vi "H_sub.vi"(4 "q 1":sgl[](array[numeric]), 5 "Id_in":i32, 6 "N 1":sgl[](array[numeric])) -> (0 "q":sgl[](array[numeric]), 2 "N":sgl[](array[numeric]))   [LabVIEW 2010]
panel:
  in  "Id_x":i32
  out "XY Graph":cluster{"q 1":sgl[], "N 1":sgl[]}[](graph)
  in  "qx":dbl
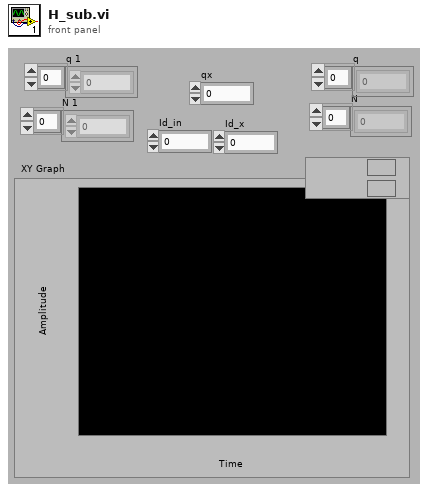
[diagram p1: front panel]
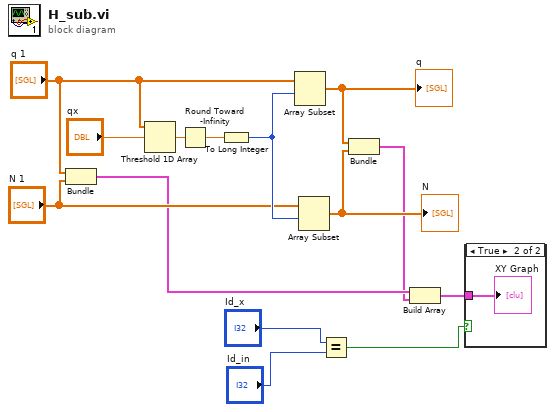
[diagram p0: block diagram]
diagram:
  n1 = Bundle("q 1"="q 1", "N 1"="N 1") -> (w6:cluster{"q 1":sgl[], "N 1":sgl[]})  [unwired: 1 in]
  n2 = Threshold 1D Array(2:"qx", 3:"q 1") -> (0:w13:sgl)  [unwired: 1 in]
  n3 = Round Toward -Infinity(1:w13) -> (0:w12:sgl)
  n4 = To Long Integer(number=w12) -> (32bit integer=w11:i32)
  n5 = Array Subset(array="q 1", index=w11) -> (w8:sgl[])  [unwired: 1 in]
  "q" <- w8
  n6 = Array Subset(array="N 1", index=w11) -> (w7:sgl[])  [unwired: 1 in]
  "N" <- w7
  n7 = Equal?(x="Id_x", y="Id_in") -> (x = y?=w1:bool)
  n8 = Bundle(w8, w7) -> (w5:cluster{sgl[], sgl[]})  [unwired: 1 in]
  n9 = Build Array(w6, w5) -> (w4:cluster{"q 1":sgl[], "N 1":sgl[]}[])
  n10 = case shown="True" w1 {
    tunnel: w4 -> [_ w15]
    frame False {
    }
    frame True {
      "XY Graph" <- w15
    }
  }
